vi "Actor Core.vi"(8 "error in":errorcluster, 11 "Measure Object in":refnum<class "Spectrum Recorder too.lvclass">) -> (0 "error out":errorcluster, 3 "Actor out":refnum<class "Actor.lvclass">)   [LabVIEW 2016, in "Spectrum Recorder too.lvclass"]
doc: "Spectrum Recorder module sweeps frequency and records complex response using Red Pitaya"
uses:
  Spectrum Recorder too.lvclass
  C:/github/LabActor/Template Module/Template Module.lvclass
  C:/Program Files/National Instruments/LabVIEW 2016/vi.lib/ActorFramework/Actor/Actor.lvclass
  <vilib>/ActorFramework/Actor/Actor.lvclass
  NHMFL_Core/Libraries/Red Pitaya/RP Core/Red Pitaya Transceiver Driver/Spectrum Configuration.ctl
  Spectrum Recorder too.lvclass/Spectrum Recorder too.ctl
  Template Module/Template Module.lvclass/Template Module.ctl
  <vilib>/ActorFramework/Actor/Actor.lvclass/Actor.ctl
  Plots/Plot types.ctl
  Controllers/Application Controller Messages/Open Waveform File Plot Msg/Open Waveform File Plot Msg.lvclass/Open Waveform File Plot Msg.ctl
  <vilib>/ActorFramework/Message Enqueuer/Message Enqueuer.lvclass/Message Enqueuer.ctl
  Template Module/Read stop event.vi
  <vilib>/ActorFramework/Message Enqueuer/Enqueue.vi
  Controllers/Application Controller Messages/Open Waveform File Plot Msg/Open Waveform File Plot Msg.lvclass
  C:/Program Files/National Instruments/LabVIEW 2016/vi.lib/ActorFramework/Message/Message.lvclass
  <vilib>/ActorFramework/Message Priority Queue/Priority Enqueue.vi
  Instrument Actor/Instrument Actor.lvclass
panel:
  in  "Fine regions' centers":dbl[](array[numeric]) format="%#_4p"
  out "Sweep duration":dbl format="%#_gs"
  out "Name":string
  in  "View XY Plot":bool
  out "Spectrum file":path caption="Spectrum File"
  out "Spectrum plot":cluster{dbl[], dbl[]}[](graph)
  in  "Configuration":T1={"Start frequency"=500000.0, "End frequency"=2000000.0, "Coarse step"=100.0, "Step duration"=0.004, "Red Pitaya address"="192.168.1.100", "Open plot \non start"=TRUE, "Regions width"=2000.0, "Fine step"=10.0, "Pause between scans"=0.0, "Clear rgs on start"=FALSE, "Output amplitude"=1.0, "Append measurements"=[]} {"Output amplitude" min=0.0 max=1.0 step=0.1 format="%#_6pV"; "Pause between scans" format="%#_6ps"; "Fine step" min=0.001 format="%#_6pHz"; "Regions width" format="%#_6pHz"; "Step duration" format="%#_6ps"; "Coarse step" format="%#_6pHz"; "End frequency" format="%#_6pHz"; "Start frequency" format="%#_6pHz"}
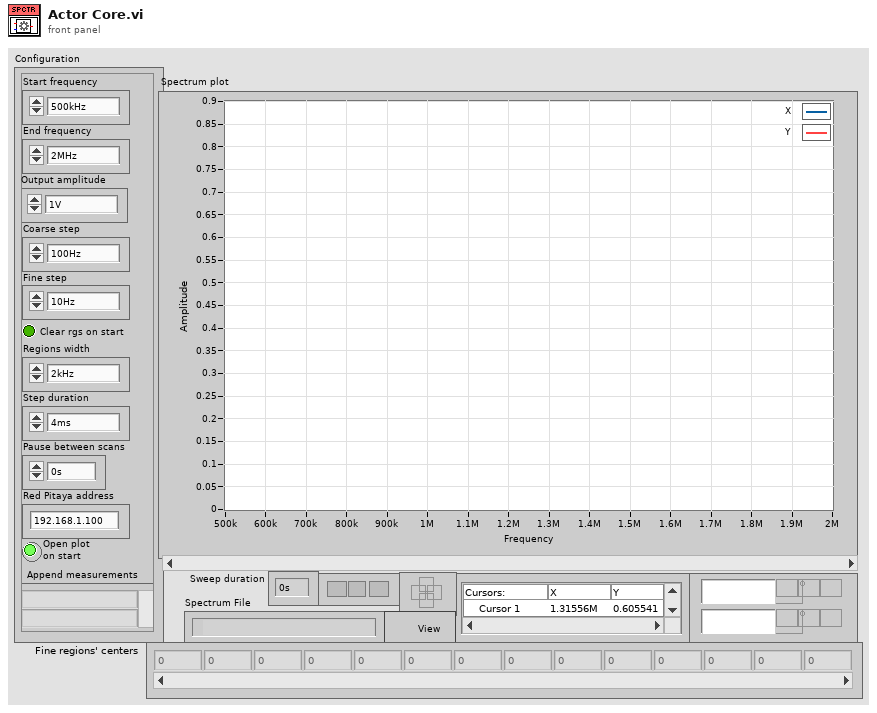
[diagram p1: front panel]
types:
  T1 = typedef "Spectrum Configuration.ctl" = cluster{"Start frequency":dbl, "End frequency":dbl, "Coarse step":dbl, "Step duration":dbl, "Red Pitaya address":string, "Open plot \non start":bool, "Regions width":dbl, "Fine step":dbl, "Pause between scans":dbl, "Clear rgs on start":bool, "Output amplitude":dbl, "Append measurements":string[]}
  T2 = typedef "Plot types.ctl" = enum16{"Waveform Plot", "XY Plot", "Full XY"}
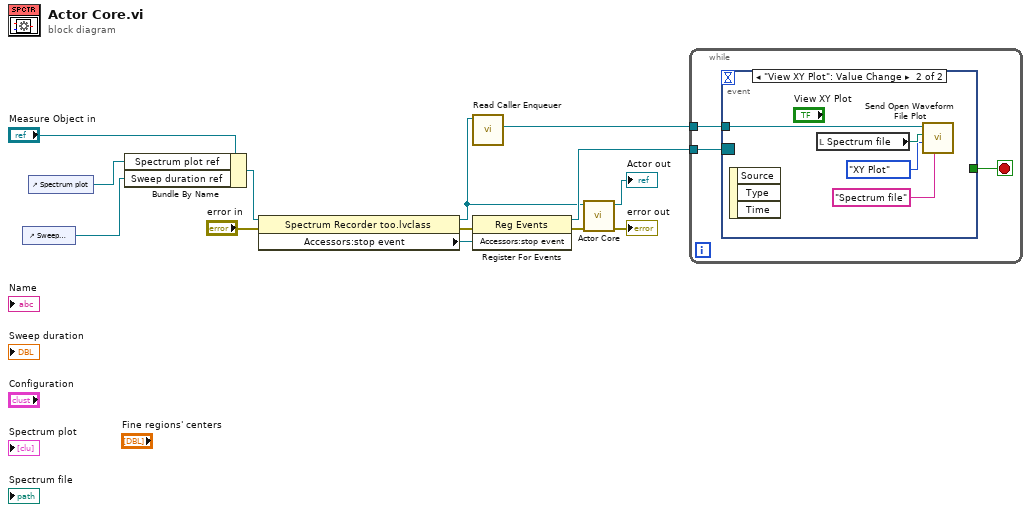
[diagram p0: block diagram]
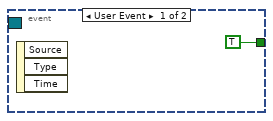
[diagram p2: hidden frame]
diagram:
  n1 = control-ref of="Sweep duration"() -> (w1:refnum<vi>)
  n2 = control-ref of="Spectrum plot"() -> (w10:refnum<vi>)
  n3 = Bundle By Name(cluster="Measure Object in", "Spectrum plot ref"=w10, "Sweep duration ref"=w1) -> (w9:refnum<class "Spectrum Recorder too.lvclass">)
  n4 = property class="Spectrum Recorder too.lvclass"(reference=w9, error in="error in") -> (reference out=w4:refnum<class "Spectrum Recorder too.lvclass">, error out=w8:errorcluster, "Accessors:stop event"=w2:refnum<user-event>)
  n5 = call <vilib>:"Read Caller Enqueuer.vi"("Actor"=w4) -> ("Caller Enqueuer"=w3:refnum<class "Message Enqueuer.lvclass">)  [unwired: 10 in]
  n6 = register-events(error in=w8, w2) -> (reference out=w5:refnum<event-registration>, error out=w6:errorcluster)  [unwired: 1 in]
  n7 = call-parent "Actor Core.vi"("error in"=w6, "Measure Object in"=w4) -> ("error out"=→"error out":errorcluster, "Actor out"=→"Actor out":refnum<class "Actor.lvclass">)  [unwired: 8 in]
  n8 = while {
    tunnel: w5 -> [w16]
    tunnel: w3 -> [w14]
    stop <- w15 stop-if-true
    n9 = event shown="[1] \"View XY Plot\": Value Change" {
      selector: w16 -> [_ _]
      dyn-events: _ -> [_ _]
      timeout: _ -> [_ _]
      tunnel: [TRUE _] -> w15
      tunnel: w14 -> [_ w21]
      event User Event {
        n10 = event-data() -> ()  [unwired: 1 in, 3 out]
      }
      event "View XY Plot": Value Change {
        n11 = event-data() -> ()  [unwired: 1 in, 3 out]
        n12 = local read "Spectrum file"() -> (w20:path)
        n13 = call "Send Open Waveform File Plot.vi"("Plot group"="Spectrum file", "Plot type"=Plot_types."XY Plot", "File Path Control"=w20, "Message Enqueuer"=w21) -> ()  [unwired: 6 in, 2 out]
      }
    }
  }
